vi "04TRM800_GetMPH.vi"(8 "error in (no error)":errorcluster, 11 "Initialize":enum16{"Initialize", "GetMPH"}(ring)) -> (0 "error out":errorcluster, 3 "MPH":i32)   [LabVIEW 2020]
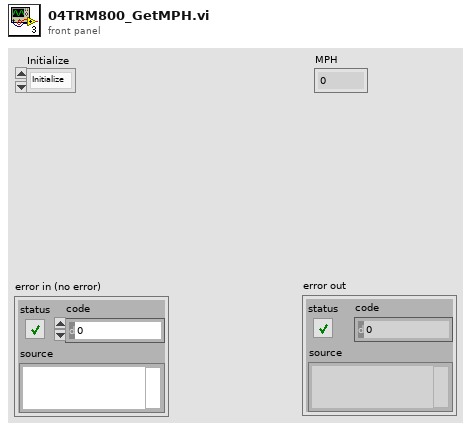
[diagram p1: front panel]
types:
  T1 = cluster{"NextChange":u32, "MPH":i32, "Stopping?":bool}
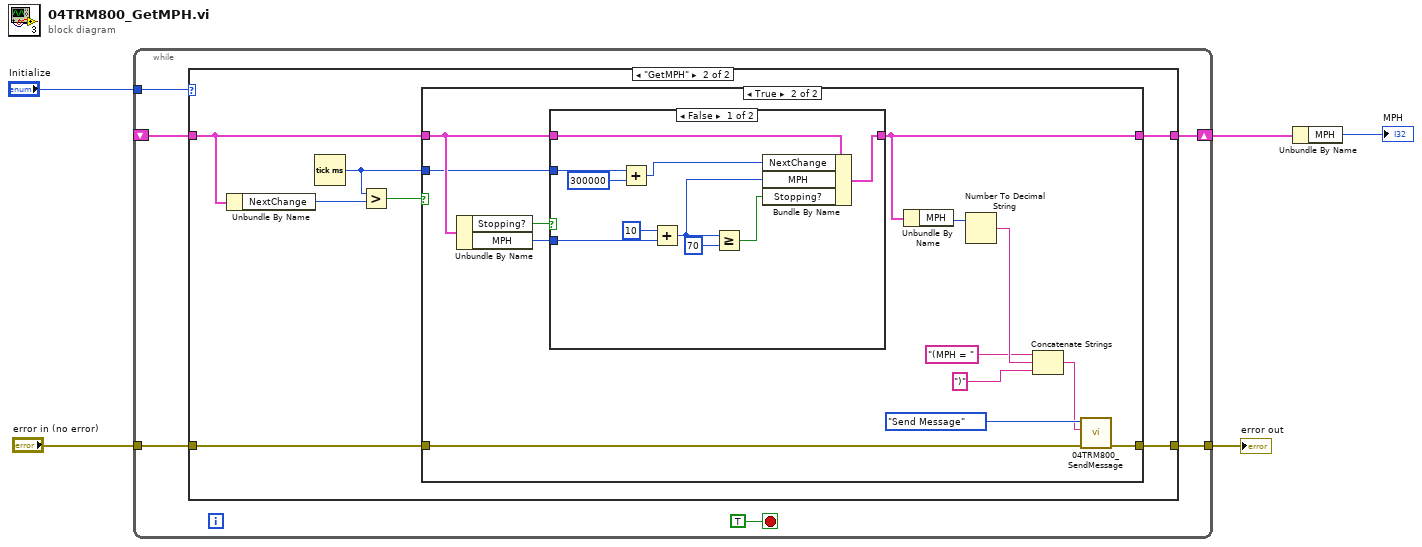
[diagram p0: block diagram]
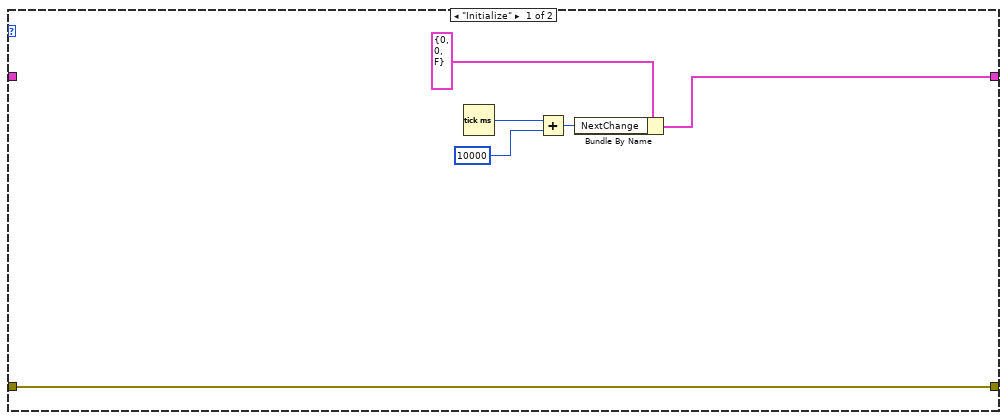
[diagram p2: hidden frame]
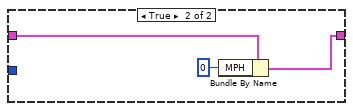
[diagram p4: hidden frame]
diagram:
  n1 = while {
    tunnel: "error in (no error)" -> [w8]
    tunnel: [w9] -> w4
    tunnel: "Initialize" -> [w10]
    shift-right: [w7] -> w2
    shift-left: _ -> [w6]
    stop <- TRUE stop-if-true
    n2 = case shown="\"GetMPH\"" w10 {
      tunnel: [w17 w21] -> w9
      tunnel: w8 -> [w17 w22]
      tunnel: [w15 w23] -> w7
      tunnel: w6 -> [_ w19]
      frame "Initialize" {
        n3 = Tick Count (ms)() -> (millisecond timer value=w14:u32)
        n4 = Add(x=w14, y=u32 10000) -> (x+y=w12:u32)
        n5 = Bundle By Name(cluster=T1 {"NextChange"=0, "MPH"=0, "Stopping?"=FALSE}, "NextChange"=w12) -> (w15:T1)
      }
      frame "GetMPH" {
        n6 = Unbundle By Name(w19) -> ("NextChange"=w18:u32)
        n7 = Tick Count (ms)() -> (millisecond timer value=w20:u32)
        n8 = Greater?(x=w20, y=w18) -> (0:w24:bool)
        n9 = case shown="True" w24 {
          tunnel: w20 -> [_ w37]
          tunnel: [w25 w35] -> w23
          tunnel: w22 -> [w26 w32]
          tunnel: [w26 w33] -> w21
          tunnel: w19 -> [w25 w39]
          frame False {
          }
          frame True {
            n10 = Unbundle By Name(w39) -> ("Stopping?"=w38:bool, "MPH"=w36:i32)
            n11 = case shown="False" w38 {
              tunnel: w39 -> [w49 w52]
              tunnel: [w48 w50] -> w35
              tunnel: w37 -> [w47 _]
              tunnel: w36 -> [w44 _]
              frame False {
                n12 = Add(x=w47, y=u32 300000) -> (x+y=w45:u32)
                n13 = Add(x=10, y=w44) -> (x+y=w42:i32)
                n14 = Greater Or Equal?(x=w42, y=70) -> (x >= y?=w41:bool)
                n15 = Bundle By Name(cluster=w49, "NextChange"=w45, "MPH"=w42, "Stopping?"=w41) -> (w48:T1)
              }
              frame True {
                n16 = Bundle By Name(cluster=w52, "MPH"=0) -> (w50:T1)
              }
            }
            n17 = Unbundle By Name(w35) -> ("MPH"=w34:i32)
            n18 = Number To Decimal String(number=w34) -> (decimal integer string=w31:string)  [unwired: 1 in]
            n19 = Concatenate Strings("(MPH = " ("string"), w31, ")" ("string")) -> (w29:string)
            n20 = call "04TRM800_SendMessage.vi"("error in (no error)"=w32, "String"=w29, "Enum"=enum16{"Initialize", "Send Message"}."Send Message") -> ("error out"=w33:errorcluster)  [unwired: 8 in]
          }
        }
      }
    }
  }
  "error out" <- w4
  n21 = Unbundle By Name(w2) -> ("MPH"=→"MPH":i32)
